vi "PrepareToLongRangeComm.vi"(8 "Error In":errorcluster, 11 "BB-Series in":refnum<class "BB-Series.lvclass">) -> (0 "Error Out":errorcluster, 3 "BB-Series out":refnum<class "BB-Series.lvclass">)   [LabVIEW 2021, in "BB-Series.lvclass"]
uses:
  BB-Series.lvclass
  Write SecurityKey.vi
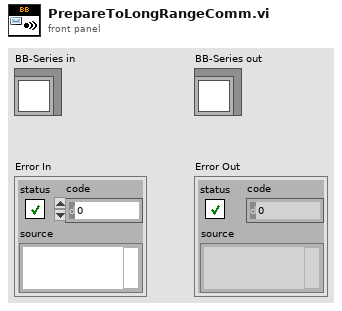
[diagram p1: front panel]
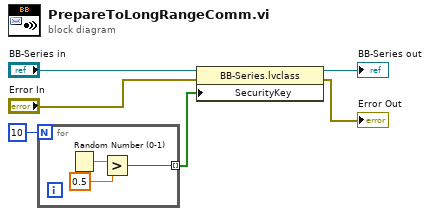
[diagram p0: block diagram]
diagram:
  n1 = for {
    N: 10 -> [_]
    tunnel: [w7] -> w4 mode=indexing
    n2 = Random Number (0-1)() -> (number: 0 to 1=w9:dbl)
    n3 = Greater?(x=w9, y=0.5) -> (0:w7:bool)
  }
  n4 = property class="BB-Series.lvclass"(reference="BB-Series in", error in="Error In", "SecurityKey"=w4) -> (reference out=→"BB-Series out":refnum<class "BB-Series.lvclass">, error out=→"Error Out":errorcluster)
